vi "Set-Get Calling VI Process ID.vi"(6 "Set/Get (F)":bool, 8 "Error In":errorcluster, 11 "ProcessID":u32) -> (0 "Error Out":errorcluster, 3 "ProcessID":u32)   [LabVIEW 2021, in "Notebook.lvlib"]
uses:
  Notebook.lvlib
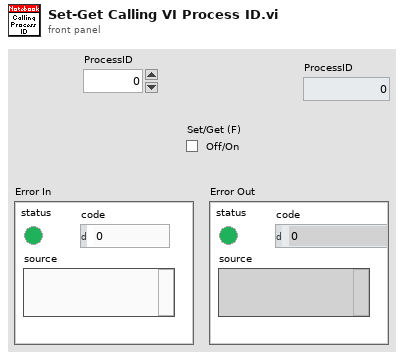
[diagram p1: front panel]
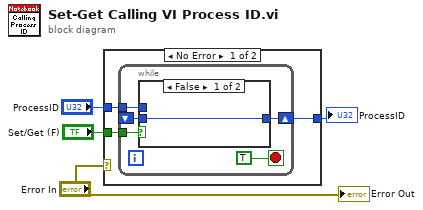
[diagram p0: block diagram]
diagram:
  n1 = case shown="No Error" "Error In" {
    tunnel: "Set/Get (F)" -> [w7 _]
    tunnel: "ProcessID" -> [w6 w15]
    tunnel: [w5 w15] -> w2
    frame No Error {
      n2 = while {
        tunnel: w7 -> [w11]
        tunnel: w6 -> [w10]
        shift-right: [w9] -> w5
        shift-left: _ -> [w8]
        stop <- TRUE stop-if-true
        n3 = case shown="False" w11 {
          tunnel: w10 -> [_ w14]
          tunnel: [w13 w14] -> w9
          tunnel: w8 -> [w13 _]
          frame False {
          }
          frame True {
          }
        }
      }
    }
    frame Error {
    }
  }
  "ProcessID" <- w2
  "Error Out" <- "Error In"
